vi "Paste Command into Command Window.vi"(7 "command":string, 8 "error in (no error)":errorcluster, 11 "hWnd":u32) -> (0 "error out":errorcluster)   [LabVIEW 2013]
uses:
  USER32.DLL
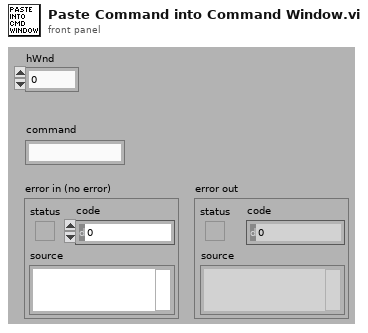
[diagram p1: front panel]
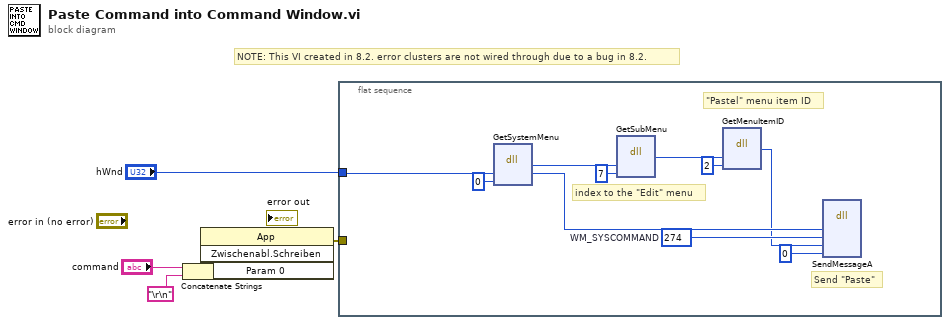
[diagram p0: block diagram]
diagram:
  # "NOTE: This VI created in 8.2. error clusters are not wired through due to a bug in 8.2."
  n1 = Concatenate Strings("command", "\r\n") -> (w2:string)
  n2 = invoke class="App" method="Zwischenabl.Schreiben"("Param 0"=w2) -> (error out=w3:errorcluster)  [unwired: 3 in, 3 out]
  n3 = flat-sequence {
    tunnel: "hWnd" -> [w6]
    tunnel: w3 -> [_]
    frame #0 {
      w11 = u32 274  # WM_SYSCOMMAND
      # "\"Pastel\" menu item ID"
      # "Send \"Paste\""
      # "index to the \"Edit\" menu"
      n4 = dll-call lib="USER32.DLL" fn="GetSystemMenu"("hWnd"=w6, "bRevert"=0) -> ("hMenu"=w14:i32, "hWnd"=w12:u32)  [unwired: 4 in, 2 out]
      n5 = dll-call lib="USER32.DLL" fn="GetSubMenu"("hMenu"=w14, "nPos"=7) -> ("hMenu"=w10:i32)  [unwired: 5 in, 2 out]
      n6 = dll-call lib="USER32.DLL" fn="GetMenuItemID"("hMenu"=w10, "nPos"=2) -> ("itemID"=w8:i32)  [unwired: 5 in, 2 out]
      n7 = dll-call lib="USER32.DLL" fn="SendMessageA" label="SendMessage"("hWnd"=w12, "msg"=w11, "wParam"=w8, "lParam"=0) -> ()  [unwired: 8 in, 2 out]
    }
  }
